vi "Login Tubes.vi"(8 "error in (no error)":errorcluster, 11 "connection information":path=path "D:/TUBES_SCADA_FIX/database.udl") -> (0 "error out":errorcluster, 1 "Role":string, 2 "User":string, 3 "Cancel":bool)   [LabVIEW 2025]
uses:
  <vilib>/Alab Technologies/AES Crypto/Public VIs/String to Array.vi
  <vilib>/Alab Technologies/AES Crypto/Public VIs/Array to String.vi
  <vilib>/addons/database/Connection.llb/DB Tools Open Connec (Path).vi
  <vilib>/addons/database/NI_Database_API.lvlib
  <vilib>/Alab Technologies/AES Crypto/AES Crypto.lvlib
panel:
  out "Output string (hex)":string
  out "Hasil Query 2":string
  out "error out 4":errorcluster
  out "Password":string
  out "error out 3":errorcluster
  out "Hasil Query":string
  in  "Tab Control":enum32{"Page 1", "Page 2", "Page 3"}(tab)
  in  "Password":string
  in  "Username":string
  in  "Login":bool
  in  "Cancel":bool
  in  "stop":bool
  in  "Lupa Password":bool
  out "error out 2":errorcluster
  in  "Multicolumn Listbox":i32(listbox)
  in  "Password Baru":string
  in  "Role":string
  in  "Username":string
  in  "Set Password":bool caption="Lupa Password"
  # "PAGE LOGIN"
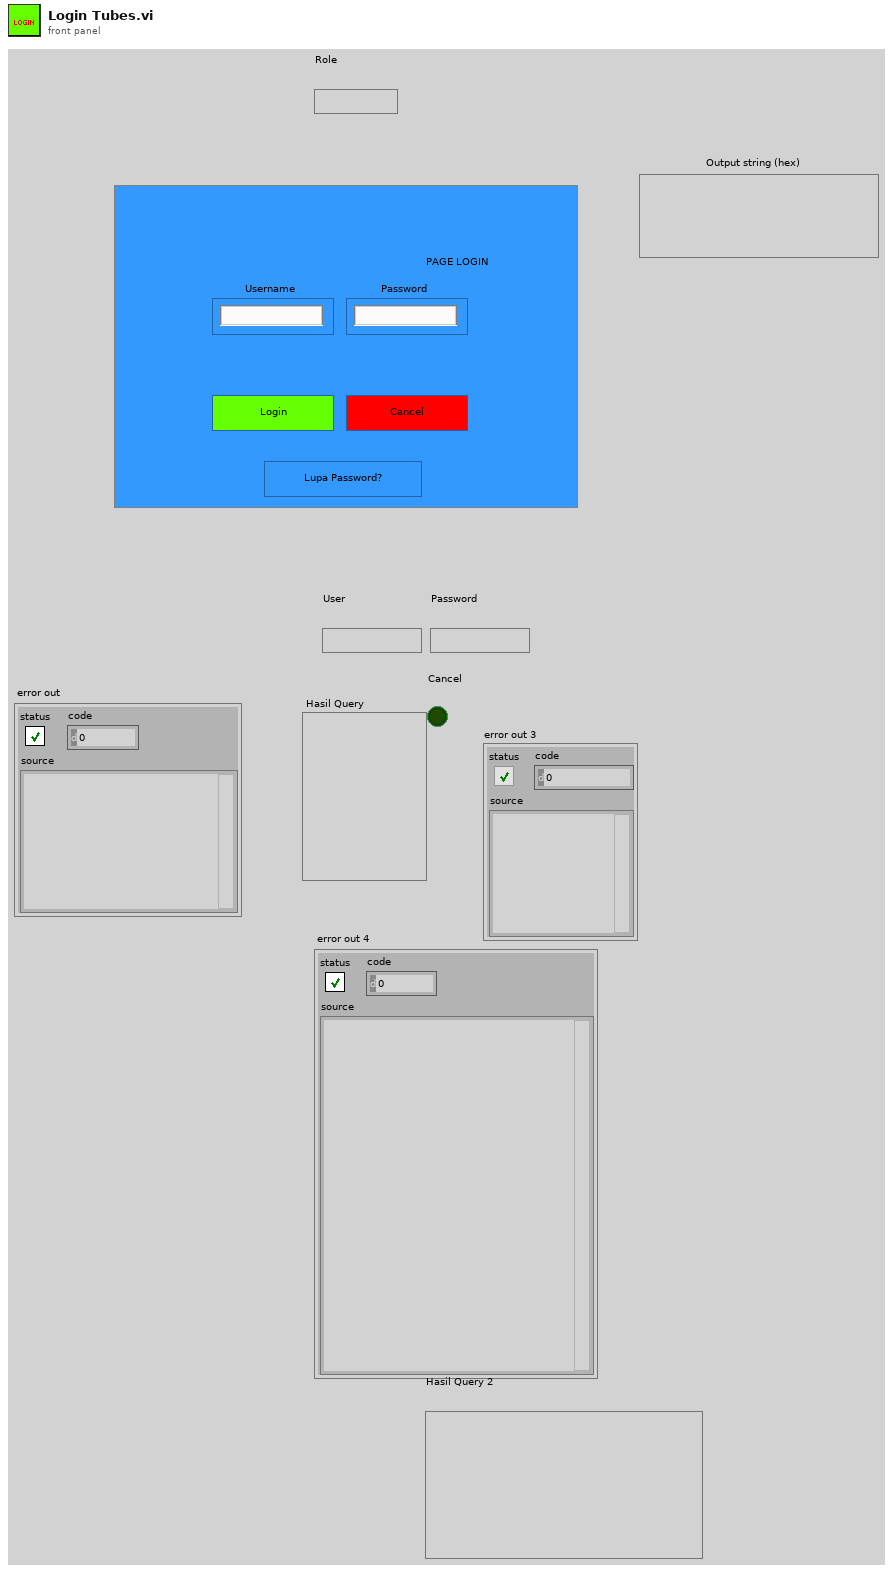
[diagram p1: front panel]
types:
  T1 = typedef "NI_Database_API.lvlib/Conn ObjectReference.ctl" = refnum<k1>
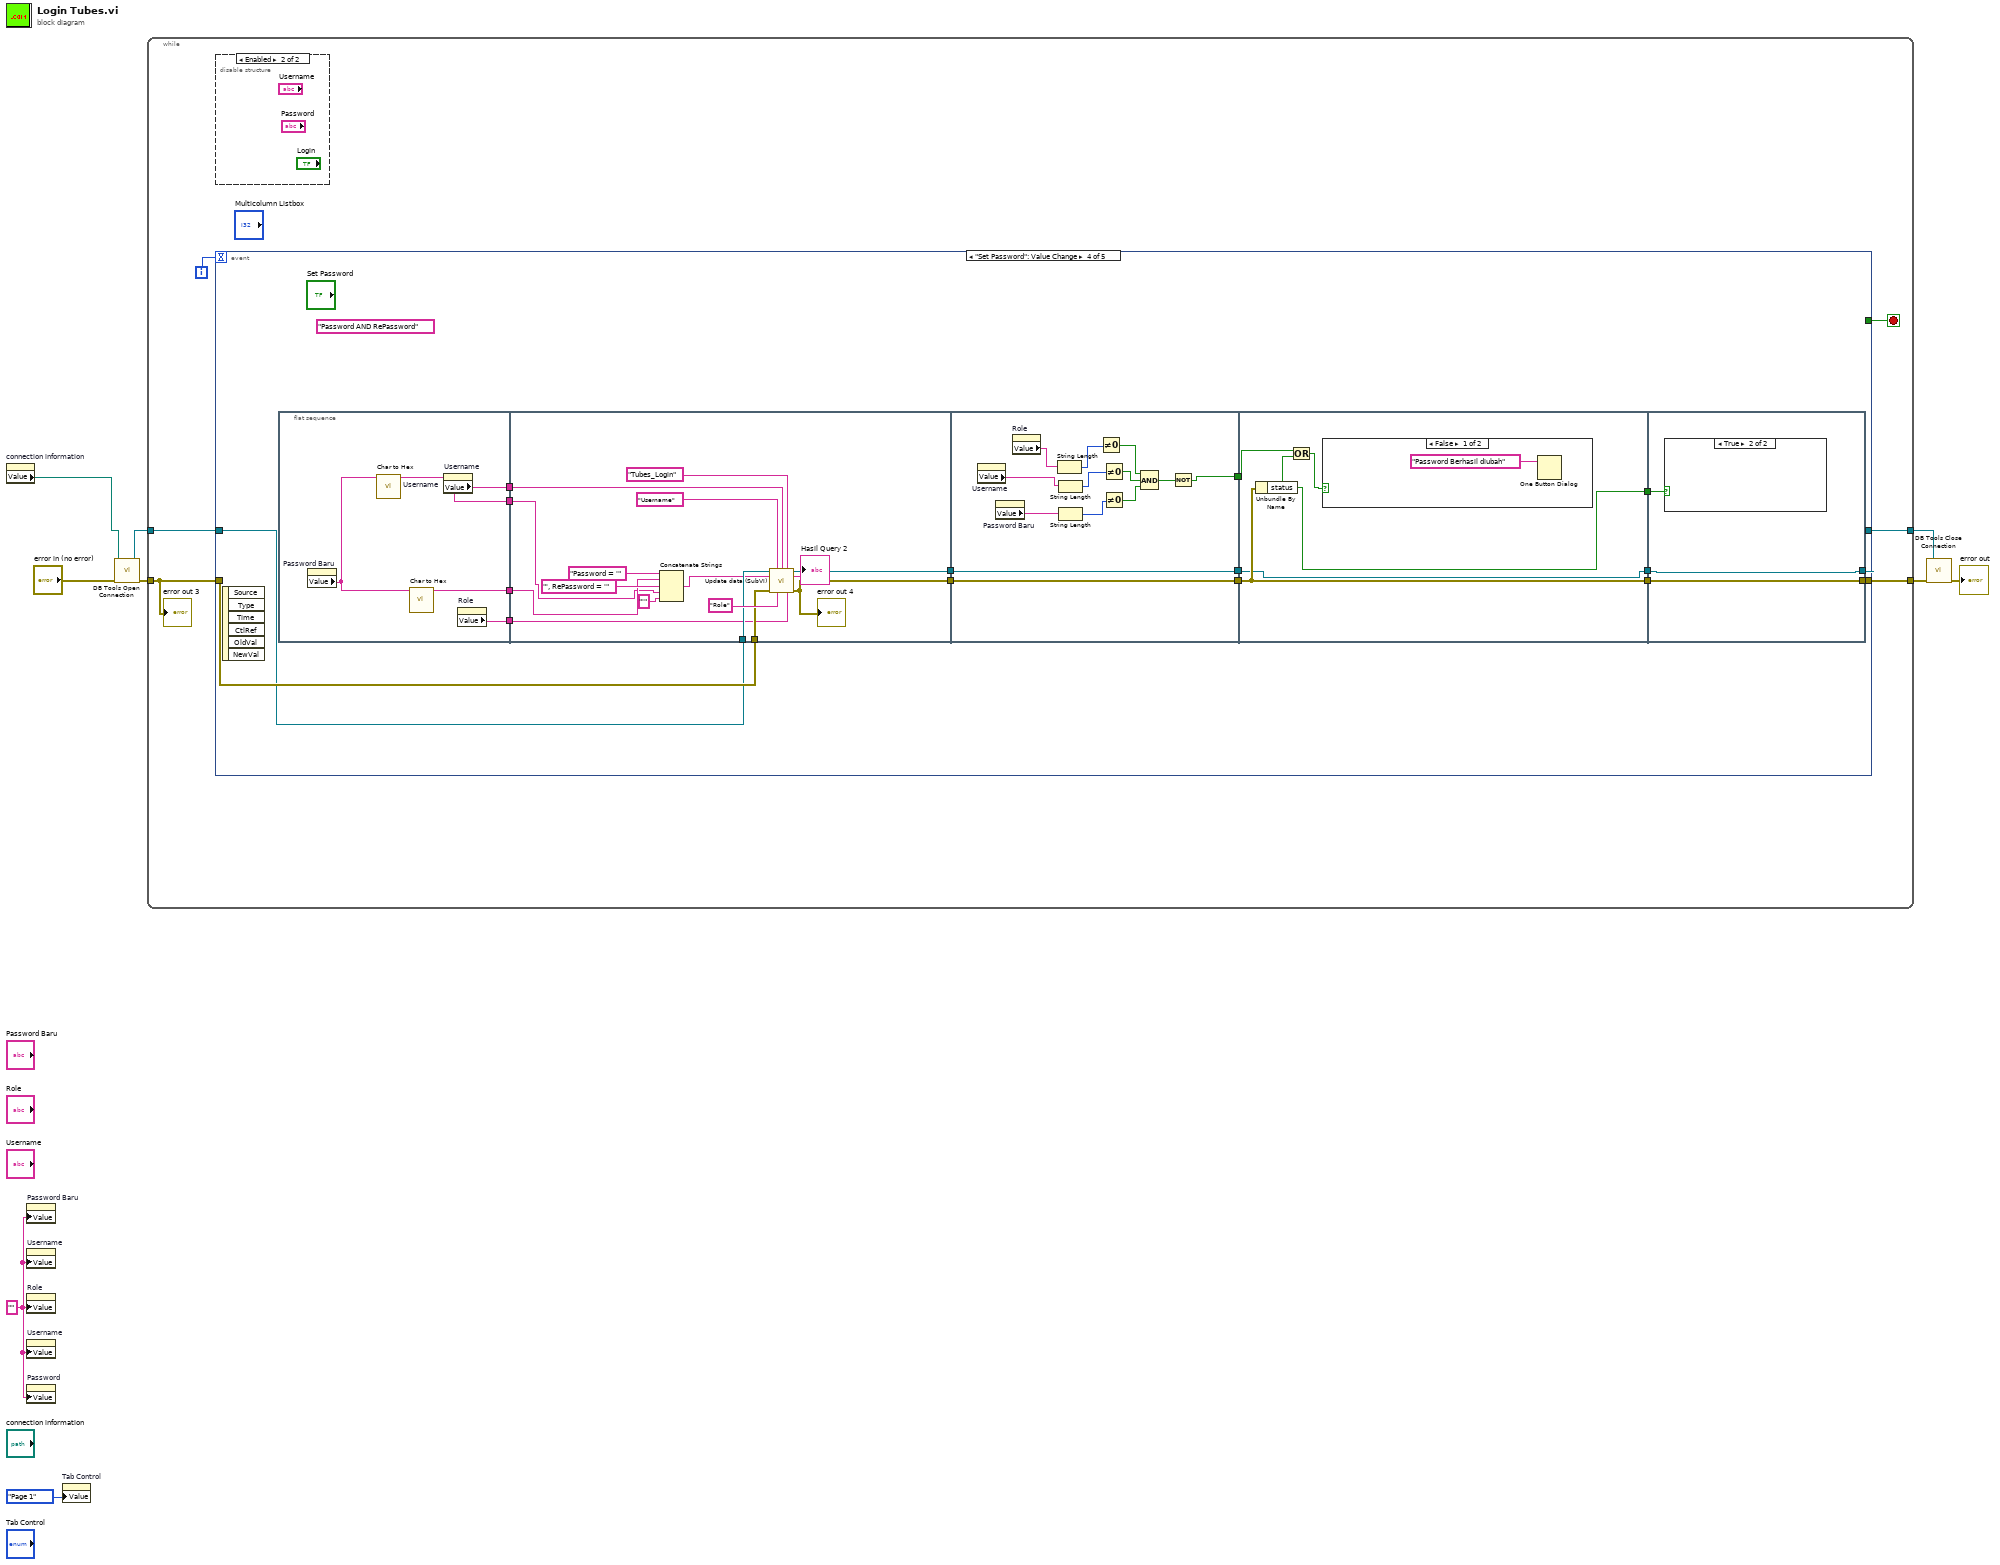
[diagram p0: block diagram]
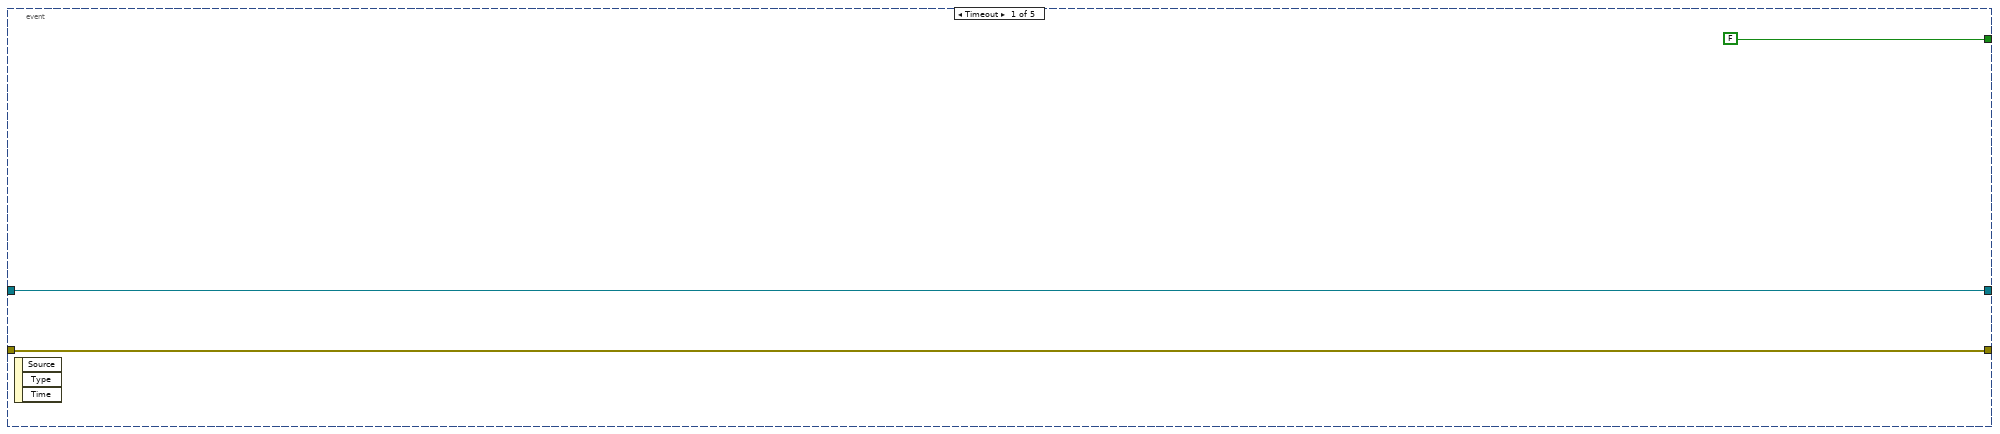
[diagram p3: hidden frame]
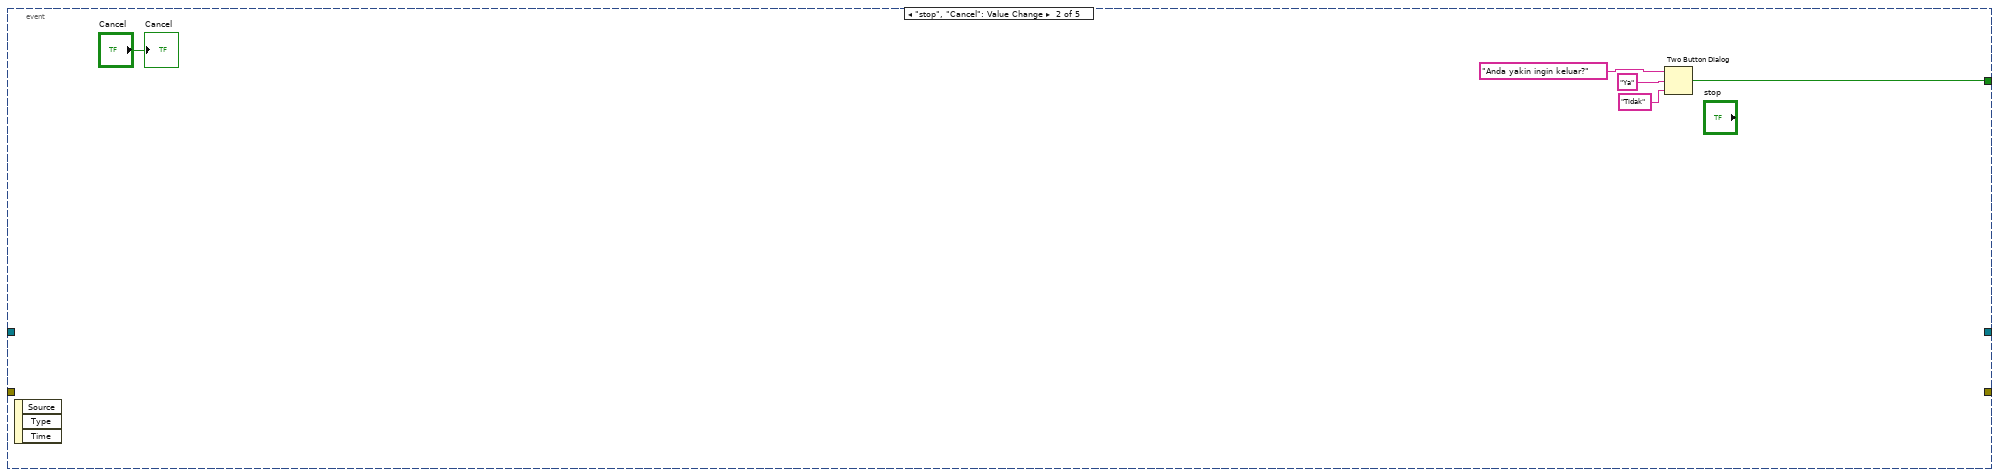
[diagram p4: hidden frame]
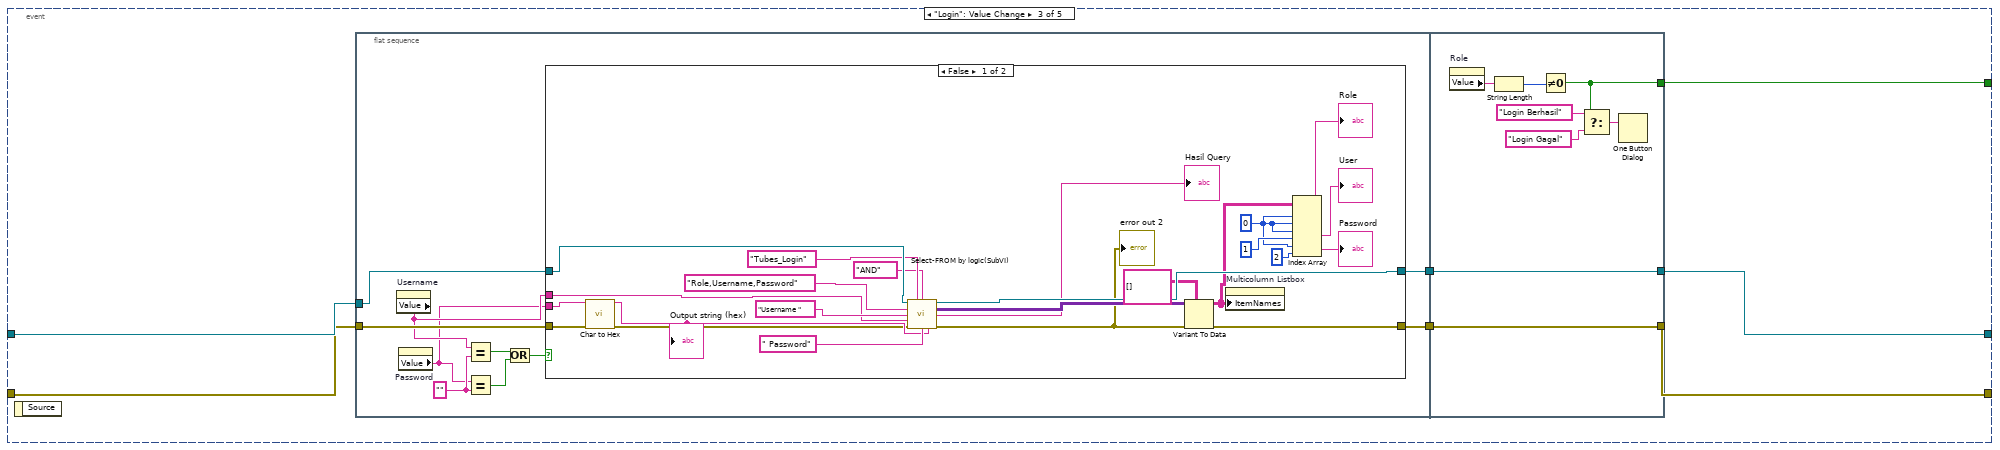
[diagram p5: hidden frame]
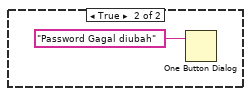
[diagram p7: hidden frame]
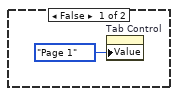
[diagram p8: hidden frame]
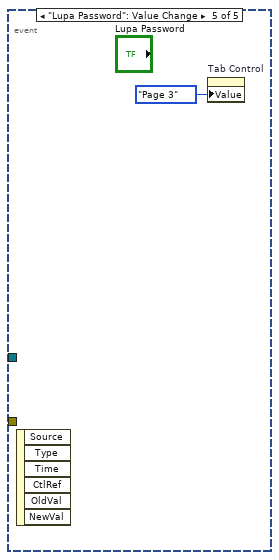
[diagram p9: hidden frame]
diagram:
  w1 = ""
  n1 = property on="connection information" class="Path"() -> ("Value"=w3:path)  [unwired: 2 in, 2 out]
  n2 = property on="Password Baru" class="Str"("Value"=w1) -> ()  [unwired: 2 in, 2 out]
  n3 = property on="Username" class="Str"("Value"=w1) -> ()  [unwired: 2 in, 2 out]
  n4 = property on="Role" class="Str"("Value"=w1) -> ()  [unwired: 2 in, 2 out]
  n5 = property on="Username" class="Str"("Value"=w1) -> ()  [unwired: 2 in, 2 out]
  n6 = property on="Password" class="Str"("Value"=w1) -> ()  [unwired: 2 in, 2 out]
  n7 = property on="Tab Control" class="TabCtl (strict)"("Value"=enum32{"Page 1", "Page 2"}."Page 1" ("Tab Control")) -> ()  [unwired: 2 in, 2 out]
  n8 = call-poly <vilib>:"DB Tools Open Connection.vi"("error in (no error)"="error in (no error)", "connection information"=w3) -> ("error out"=w7:errorcluster, "connection reference"=w9:T1)  [unwired: 6 in]
  n9 = while {
    tunnel: w9 -> [w14]
    tunnel: [w13] -> w8
    tunnel: w7 -> [w12]
    tunnel: [w11] -> w6
    i -> [w15]
    stop <- w10 stop-if-true
    n10 = disable-structure shown="Enabled" {
      frame Disabled {
      }
      frame Enabled {
      }
    }
    n11 = event shown="[3] \"Set Password\": Value Change" {
      selector: _ -> [_ _ _ _ _]
      dyn-events: _ -> [_ _ _ _ _]
      timeout: w15 -> [_ _ _ _ _]
      tunnel: w14 -> [w18 _ w30 w88 _]
      tunnel: [w18 _ w25 w87 _] -> w13
      tunnel: w12 -> [w17 _ w29 w89 _]
      tunnel: [w17 _ w28 w86 _] -> w11
      tunnel: [FALSE ("T button?") w20 w24 _ _] -> w10
      event Timeout {
        n12 = event-data() -> ()  [unwired: 1 in, 3 out]
      }
      event "stop", "Cancel": Value Change {
        n13 = event-data() -> ()  [unwired: 1 in, 3 out]
        n14 = Two Button Dialog(message="Anda yakin ingin keluar?", 1:"Tidak" ("F button name (\"Cancel\")"), 2:"Ya" ("T button name (\"OK\")")) -> (T button?=w20:bool)
        "Cancel" <- "Cancel"
      }
      event "Login": Value Change {
        n15 = event-data() -> ()  [unwired: 1 in, 1 out]
        n16 = flat-sequence {
          tunnel: w30 -> [w40]
          tunnel: w29 -> [w38]
          tunnel: [w39] -> w27
          tunnel: [w37] -> w26
          tunnel: [w73] -> w28
          tunnel: [w74] -> w25
          tunnel: w27 -> [w74]
          tunnel: w26 -> [w73]
          tunnel: [w67] -> w24
          frame #0 {
            w34 = "" ("y")
            n17 = property on="Username" class="Str"() -> ("Value"=w32:string)  [unwired: 2 in, 2 out]
            n18 = property on="Password" class="Str"() -> ("Value"=w31:string)  [unwired: 2 in, 2 out]
            n19 = Equal?(x=w32, y=w34) -> (x = y?=w35:bool)
            n20 = Equal?(x=w31, y=w34) -> (x = y?=w36:bool)
            n21 = Or(x=w35, y=w36) -> (x .or. y?=w33:bool)
            n22 = case shown="False" w33 {
              tunnel: w40 -> [w64 w65]
              tunnel: [w63 w65] -> w39
              tunnel: w38 -> [w47 w66]
              tunnel: [w61 w66] -> w37
              tunnel: w32 -> [w50 _]
              tunnel: w31 -> [w49 _]
              frame False {
                w43 = 0 ("index (row)")
                n23 = call <vilib>:"Char to Hex.vi"("Input string (char)"=w49, "error in (no error)"=w47) -> ("Output string (hex)"=w48:string, "error out"=w46:errorcluster)  [unwired: 12 in]
                "Output string (hex)" <- w48
                n24 = call "Select-FROM by logic(SubVI).vi"("connection reference"=w64, "TABLE"="Tubes_Login", "Logic data"="AND", "COLOUM 1"="Role,Username,Password", "COLOUM Data 1"="Username " ("COLOUM Data"), "Nilai 1"=w50, "error in (no error)"=w46, "COLOUM Data 2"=" Password", "Nilai 2"=w48) -> ("connection reference 2"=w63:T1, "recordset data"=w62:variant[][], "Hasil Query"=→"Hasil Query":string, "error out"=w58:errorcluster)  [unwired: 2 in, 1 out]
                "error out 2" <- w58
                n25 = Variant To Data(error in=w58, type=string[][] [], Variant=w62) -> (data=w60:string[][], error out=w61:errorcluster)
                n26 = property on="Multicolumn Listbox" class="MCListbox (strict)"("ItemNames"=w60) -> ()  [unwired: 2 in, 2 out]
                n27 = Index Array(array=w60, index (row) #1=w43, index (col) #1=w43, index (row) #2=w43, index (col) #2=1 ("disabled index (col)"), index (row) #3=w43, index (col) #3=2 ("disabled index (col)")) -> (element #1=→"Role":string, element #2=→"User":string, element #3=→"Password":string)
              }
              frame True {
              }
            }
          }
          frame #1 {
            n28 = property on="Role" class="Str"() -> ("Value"=w71:string)  [unwired: 2 in, 2 out]
            n29 = String Length(string=w71) -> (length=w72:i32)
            n30 = Not Equal To 0?(x=w72) -> (x != 0?=w67:bool)
            n31 = Select(t="Login Berhasil" ("message"), s=w67, f="Login Gagal" ("message")) -> (s? t:f=w70:string)
            n32 = One Button Dialog(message=w70) -> ()  [unwired: 1 in, 1 out]
          }
        }
      }
      event "Set Password": Value Change {
        (unwired) "Password AND RePassword" ("Set Kolom")
        n33 = event-data() -> ()  [unwired: 1 in, 6 out]
        n34 = flat-sequence {
          tunnel: [w95] -> w90
          tunnel: [w94] -> w83
          tunnel: [w93] -> w82
          tunnel: [w91] -> w81
          tunnel: w90 -> [w97]
          tunnel: w89 -> [w109]
          tunnel: w88 -> [w108]
          tunnel: [w107] -> w80
          tunnel: [w106] -> w78
          tunnel: w83 -> [w98]
          tunnel: w82 -> [w105]
          tunnel: w81 -> [w96]
          tunnel: w80 -> [w124]
          tunnel: [w124] -> w79
          tunnel: w78 -> [w123]
          tunnel: [w123] -> w77
          tunnel: [w112] -> w76
          tunnel: w79 -> [w129]
          tunnel: w77 -> [w128]
          tunnel: [w129] -> w85
          tunnel: [w128] -> w84
          tunnel: w76 -> [w127]
          tunnel: [w125] -> w75
          tunnel: [w133] -> w87
          tunnel: [w134] -> w86
          tunnel: w85 -> [w134]
          tunnel: w84 -> [w133]
          tunnel: w75 -> [w132]
          frame #0 {
            n35 = property on="Password Baru" class="Str"() -> ("Value"=w92:string)  [unwired: 2 in, 2 out]
            n36 = call <vilib>:"Char to Hex.vi"("Input string (char)"=w92) -> ("Output string (hex)"=w91:string)  [unwired: 13 in, 1 out]
            n37 = call <vilib>:"Char to Hex.vi"("Input string (char)"=w92) -> ("Output string (hex)"=w95:string)  [unwired: 13 in, 1 out]
            n38 = property on="Username" class="Str" props=["Value"]() -> ()  [unwired: 2 in, 3 out]
            n39 = property on="Username" class="Str"() -> ("Value"=w93:string)  [unwired: 2 in, 2 out]
            n40 = property on="Role" class="Str"() -> ("Value"=w94:string)  [unwired: 2 in, 2 out]
          }
          frame #1 {
            n41 = Concatenate Strings("Password = '" ("string"), w97, "', RePassword = '" ("string"), w96, "'" ("string")) -> (w100:string)
            n42 = call "Update data (SubVI).vi"("Refnum in"=w108, "Kolom Username"="Username", "Nilai User"=w105, "Nama Table"="Tubes_Login", "Set Kolom"=w100, "error in (no error)"=w109, "Kolom Role"="Role" ("Kolom Acuan"), "Nilai Role"=w98) -> ("Refnum out"=w106:T1, "Hasil Query"=→"Hasil Query 2":string, "error out"=w107:errorcluster)  [unwired: 5 in]
            "error out 4" <- w107
          }
          frame #2 {
            n43 = property on="Username" class="Str"() -> ("Value"=w121:string)  [unwired: 2 in, 2 out]
            n44 = property on="Password Baru" class="Str"() -> ("Value"=w120:string)  [unwired: 2 in, 2 out]
            n45 = property on="Role" class="Str"() -> ("Value"=w122:string)  [unwired: 2 in, 2 out]
            n46 = String Length(string=w122) -> (length=w118:i32)
            n47 = String Length(string=w121) -> (length=w117:i32)
            n48 = String Length(string=w120) -> (length=w114:i32)
            n49 = Not Equal To 0?(x=w118) -> (x != 0?=w116:bool)
            n50 = Not Equal To 0?(x=w117) -> (x != 0?=w115:bool)
            n51 = Not Equal To 0?(x=w114) -> (x != 0?=w119:bool)
            n52 = Compound Arithmetic op=AND(w116, w115, w119) -> (w113:bool)
            n53 = Not(x=w113) -> (.not. x?=w112:bool)
          }
          frame #3 {
            n54 = Unbundle By Name(w129) -> ("status"=w125:bool)
            n55 = Or(x=w127, y=w125) -> (x .or. y?=w126:bool)
            n56 = case shown="False" w126 {
              frame False {
                n57 = One Button Dialog(message="Password Berhasil diubah") -> ()  [unwired: 1 in, 1 out]
              }
              frame True {
                n58 = One Button Dialog(message="Password Gagal diubah") -> ()  [unwired: 1 in, 1 out]
              }
            }
          }
          frame #4 {
            n59 = case shown="True" w132 {
              frame False {
                n60 = property on="Tab Control" class="TabCtl (strict)"("Value"=enum32{"Page 1", "Page 2", "Page 3"}."Page 1" ("Tab Control")) -> ()  [unwired: 2 in, 2 out]
              }
              frame True {
              }
            }
          }
        }
      }
      event "Lupa Password": Value Change {
        n61 = event-data() -> ()  [unwired: 1 in, 6 out]
        n62 = property on="Tab Control" class="TabCtl (strict)"("Value"=enum32{"Page 1", "Page 2", "Page 3"}."Page 3" ("Tab Control")) -> ()  [unwired: 2 in, 2 out]
      }
    }
    "error out 3" <- w12
  }
  n63 = call <vilib>:"DB Tools Close Connection.vi"("error in (no error)"=w6, "connection reference"=w8) -> ("error out"=→"error out":errorcluster)  [unwired: 5 in]
